vi "CheckPasserState.vi"(8 "error in (no error)":errorcluster, 10 "GameRef":refnum<data-value>, 11 "object in":refnum<class "PositionTactic.lvclass">) -> (0 "error out":errorcluster, 2 "goToGuardPos":bool=TRUE, 3 "object out":refnum<class "PositionTactic.lvclass">)   [LabVIEW 2023, in "PositionTactic.lvclass"]
uses:
  PositionTactic.lvclass
  PositionTactic.lvclass/PositionTactic.ctl
  Robot_class/roles.ctl
  Utilities_class/Utilities.lvclass
  PrimaryAttacker_class/PrimaryAttackerRole_states.ctl
  PrimaryAttacker_class/PrimaryAttackerRole.lvclass
  Ally_class/Ally.lvclass
  Game_class/Game.lvclass
  NewSTP/NewRoles/Role_v2_class/Role_v2.lvclass
  Robot_class/Robot.lvclass
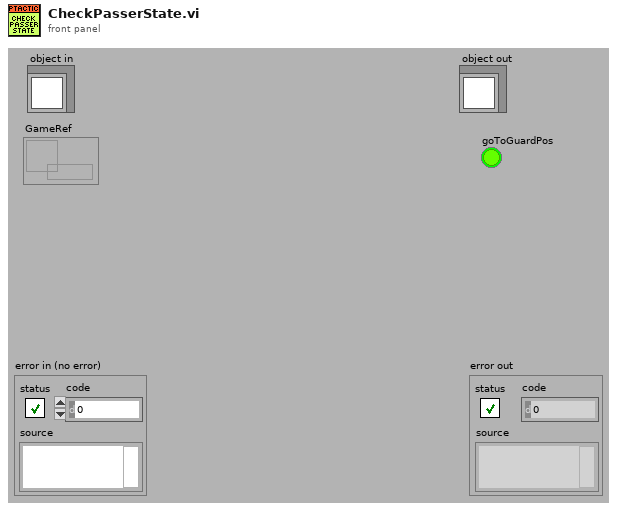
[diagram p1: front panel]
types:
  T1 = typedef "roles.ctl" = enum16{"SimpleBallPlacement", "BallPlacementAllyPasser", "BallPlacementAllyReceiver", "BallPlacementEnemy", "5Robots5th", "PassBestReceiver", "5Robots4th", "5Robots3rd", "5Robots2nd", "5Robots1st", "PassBestRobot", "WaitPass", "ABCThirdKicker", "ABCFirstKicker", "ABCSecondKicker", "Tabler", "TableFinalizer", "PrepareRollToPassRoller", "PrepareRollToPassReceiver", "SimplePassRoll", "SimplePassRollReceiver", "PenaltyDefense", "PreparePassReceiver 2", "PreparePassReceiver 1", "PassObserver", "Timeout", "Goto", "ZigZag", "None", "BallOutOfField", "DefenderArea", "Duelist", "AttackerStop", "FollowAttacker", "KeeperRole", "KickPenalty", "AttackerAimGoal", "AttackerBlock", "Marker", "Halt", "Shoot", "PassKicker", "PassReceiver", "TestRole", "PenaltyAttacker", "PrimaryAttackerRole", "SupportAttackerRole"}
  T2 = typedef "PrimaryAttackerRole.lvclass/PrimaryAttackerRole_states.ctl" = enum16{"Shoot", "PreparePass", "Pass", "Exit"}
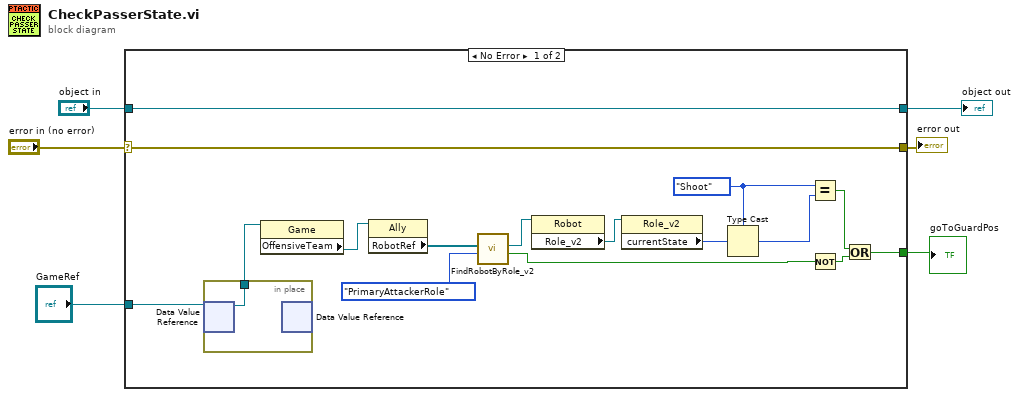
[diagram p0: block diagram]
diagram:
  n1 = case shown="No Error" "error in (no error)" {
    selector: "error in (no error)" -> [w22 w25]
    tunnel: [w22 w25] -> w5
    tunnel: [w21 w24] -> w3
    tunnel: "object in" -> [w21 w24]
    tunnel: "GameRef" -> [w10 _]
    tunnel: [w9 _] -> w1
    frame No Error {
      w12 = PrimaryAttackerRole_states."Shoot" ("Enum")
      n2 = in-place {
        in-place-border: [w23] -> w20
        n3 = in-place-dvr #1(w10) -> (w23:refnum<class "Game.lvclass">)  [unwired: 1 out]
        n4 = in-place-dvr #1() -> ()  [unwired: 1 in, 2 out]
      }
      n5 = property class="Game"(reference=w20) -> ("OffensiveTeam"=w19:refnum<class "Ally.lvclass">)  [unwired: 1 in, 2 out]
      n6 = property class="Ally"(reference=w19) -> ("RobotRef"=w18:refnum<class "Robot.lvclass">[])  [unwired: 1 in, 2 out]
      n7 = call "FindRobotByRole_v2.vi"("role"=roles."PrimaryAttackerRole", "Array"=w18) -> ("foundRobot"=w7:bool, "Robot"=w16:refnum<class "Robot.lvclass">)  [unwired: 6 in, 2 out]
      n8 = property class="Robot"(reference=w16) -> ("Role_v2"=w15:refnum<class "Role_v2.lvclass">)  [unwired: 1 in, 2 out]
      n9 = property class="Role_v2"(reference=w15) -> ("currentState"=w14:u8)  [unwired: 1 in, 2 out]
      n10 = Type Cast(type=w12, x=w14) -> (*(type *) &x=w13:T2)
      n11 = Equal?(x=w12, y=w13) -> (x = y?=w11:bool)
      n12 = Not(x=w7) -> (.not. x?=w8:bool)
      n13 = Or(x=w11, y=w8) -> (x .or. y?=w9:bool)
    }
    frame Error {
    }
  }
  "error out" <- w5
  "object out" <- w3
  "goToGuardPos" <- w1
